vi "Init Msg Output.vi"() -> (3 "Stopped Msg Output out":refnum<class "Stopped Msg Output.lvclass">)   [LabVIEW 2020, in "jettl.lvlib" / "Stopped jettl Msg.lvlib" / "Stopped Msg Output.lvlib" / "Stopped Msg Output.lvclass"]
uses:
  Stopped Msg Output.lvclass
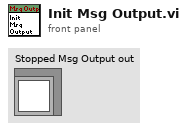
[diagram p1: front panel]
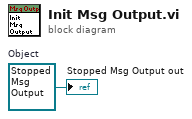
[diagram p0: block diagram]
diagram:
  w1 = refnum<class "Stopped Msg Output.lvclass"> refnum  # Object
  "Stopped Msg Output out" <- w1
